vi "SHT30.vi"() -> ()   [LabVIEW 2021]
uses:
  <vilib>/Instr/_visa.llb/VISA Configure Serial Port (Instr).vi
panel:
  out "Waveform Chart 2":dbl(graph)=76.5
  out "Waveform Chart":dbl(graph)=25.51
  out "read buffer":string="Temp *C = 25.51\t\tHum. % = 76.50\r\n"
  out "Humi (%)":dbl=76.5
  out "Temp (C)":dbl=25.51
  in  "stop":bool
  in  "baud rate (9600)":u32=115200
  in  "VISA resource name":refnum<visa-resource-name>="COM4"
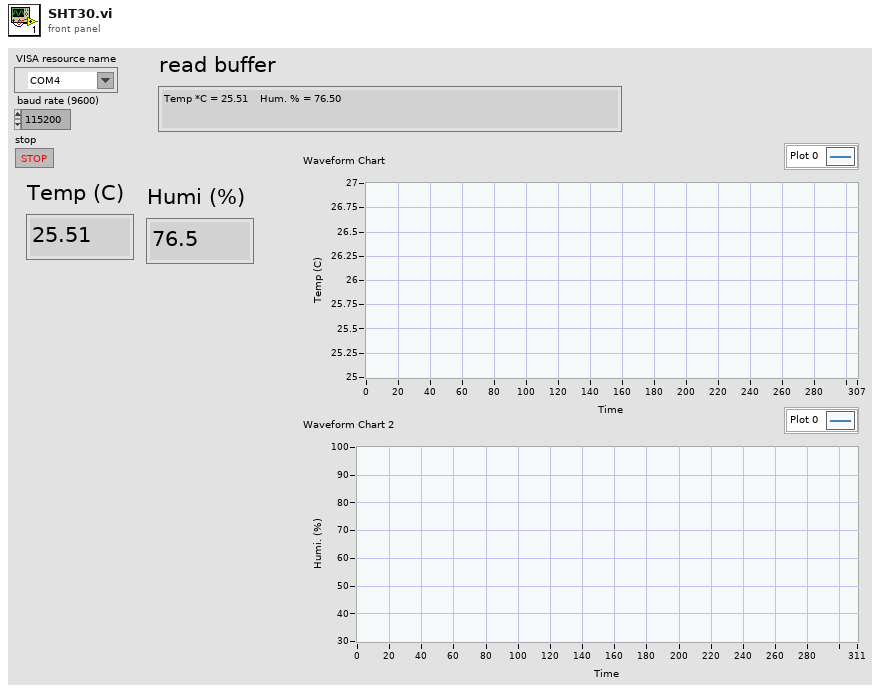
[diagram p1: front panel]
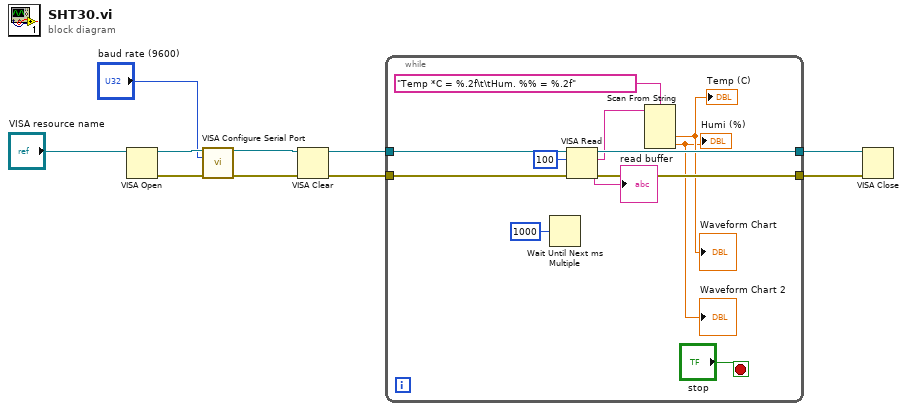
[diagram p0: block diagram]
diagram:
  n1 = VISA Open(VISA resource name="VISA resource name") -> (VISA resource name=w9:refnum<visa-resource-name>, error out=w8:errorcluster)  [unwired: 4 in]
  n2 = call-poly "VISA Configure Serial Port"("VISA resource name"=w9, "baud rate (9600)"="baud rate (9600)", "error in (no error)"=w8) -> ("VISA resource name out"=w6:refnum<visa-resource-name>, "error out"=w5:errorcluster)  [unwired: 11 in]
  n3 = VISA Clear(VISA resource name=w6, error in (no error)=w5) -> (VISA resource name out=w4:refnum<visa-resource-name>, error out=w3:errorcluster)
  n4 = while {
    tunnel: w4 -> [w21]
    tunnel: [w19] -> w2
    tunnel: w3 -> [w20]
    tunnel: [w18] -> w1
    stop <- "stop" stop-if-true
    n5 = Wait Until Next ms Multiple(millisecond multiple=u32 1000) -> ()  [unwired: 1 out]
    n6 = VISA Read(VISA resource name=w21, byte count=u32 100, error in (no error)=w20) -> (VISA resource name out=w19:refnum<visa-resource-name>, read buffer=w14:string, error out=w18:errorcluster)  [unwired: 1 out]
    "read buffer" <- w14
    n7 = Scan From String(format string="Temp *C = %.2f\t\tHum. %% = %.2f", input string=w14) -> (output 1=→"Temp (C)" →"Waveform Chart":dbl, output 2=→"Humi (%)" →"Waveform Chart 2":dbl)  [unwired: 4 in, 3 out]
  }
  n8 = VISA Close(VISA resource name=w2, error in (no error)=w1) -> ()  [unwired: 1 out]
